vi "SetAttributeViBoolean_SS-DMod_ListSeq_RF.vi"(7 "AttributeValue (Off)":bool, 8 "error in (no error)":errorcluster {"code" format="%.0x"}, 9 "AttributeID":u32(ring)=1150917 items=["SS_DIGITALMODULATION_ARB_ENABLED"=1150917, "SS_DIGITALMODULATION_ARB_EXTERNAL_TRIGGER_DELAY_ENABLED"=1150886, "SS_DIGITALMODULATION_ARB_IQADJUSTMENT_ENABLED"=1150918, "SS_DIGITALMODULATION_ARB_SEQUENCE_SYNC_ENABLED"=1150907, "SS_LISTSEQUENCER_ENABLED"=1150903, "SS_RFGENERATOR_MODULATION_AM_ENABLED"=1150927, "SS_RFGENERATOR_MODULATION_ENABLED"=1150940, "SS_RFGENERATOR_MODULATION_FM_ENABLED"=1150930, "SS_RFGENERATOR_MODULATION_PM_ENABLED"=1150932, "SS_RFGENERATOR_OUTPUT_ENABLED"=1150942, "SS_RFGENERATOR_REFERENCE_FREQUENCY_ENABLED"=1150913, "SS_RFGENERATOR_REFERENCE_POWER_ENABLED"=1150915], 10 "RepCapIdentifier":string, 11 "instrument handle":refnum<k15>) -> (0 "error out":errorcluster {"code" format="%.0x"}, 3 "instrument handle out":refnum<k15>)   [LabVIEW 2009, in "Keysight XSAn.lvlib"]
doc: "Sets a Boolean attribute from the instrument driver.\nThe following Attributes are supported:\n\nSS_DIGITALMODULATION_ARB_ENABLED\nSS_DIGITALMODULATION_ARB_EXTERNAL_TRIGGER_DELAY_ENABLED\nSS_DIGITALMODULATION_ARB_IQADJUSTMENT_ENABLED\nSS_DIGITALMODULATION_ARB_SEQUENCE_SYNC_ENABLED\nSS_LISTSEQUENCER_ENABLED\nSS_RFGENERATOR_MODULATION_AM_ENABLED\nSS_RFGENERATOR_MODULATION_ENABLED\nSS_RFGENERATOR_MODULATION_FM_ENABLED\nSS_RFGENERATOR_MODULATION_PM_ENABLED\nSS_RFGENERATOR_OUTPUT_ENABLED\nSS_RFGENERATOR_REFERENCE_FREQUENCY_ENABLED\nSS_RFGENERATOR_REFERENCE_POWER_ENABLED"
uses:
  <instrlib>/Keysight XSAn/Keysight XSAn.lvlib
  AgXSAn.dll
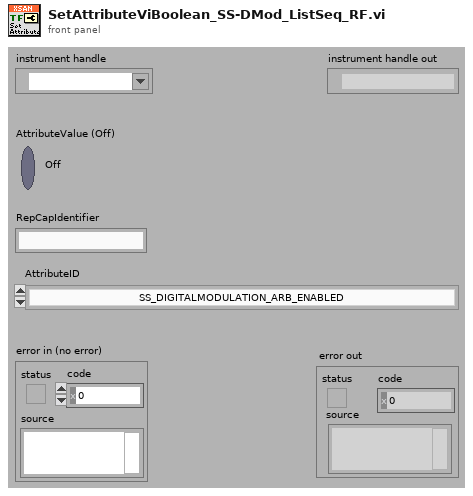
[diagram p1: front panel]
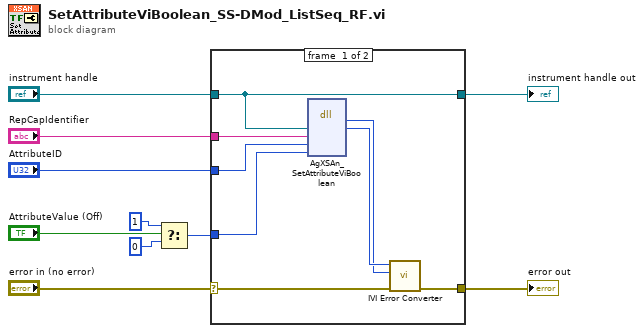
[diagram p0: block diagram]
diagram:
  n1 = Select(t=u16 1, s="AttributeValue (Off)", f=u16 0) -> (s? t:f=w3:u16)
  n2 = case shown="No Error" "error in (no error)" {
    selector: "error in (no error)" -> [w16 w20]
    tunnel: [w15 w20] -> w10
    tunnel: "instrument handle" -> [w11 w19]
    tunnel: "RepCapIdentifier" -> [w14 _]
    tunnel: "AttributeID" -> [w13 _]
    tunnel: w3 -> [w12 _]
    tunnel: [w11 w19] -> w2
    frame #0 {
      n3 = dll-call lib="AgXSAn**.dll" fn="AgXSAn_SetAttributeViBoolean"("Vi"=w11, "RepCapIdentifier"=w14, "AttributeID"=w13, "AttributeValue"=w12) -> ("return type"=w17:i32, "Vi"=w18:u32)  [unwired: 6 in, 2 out]
      n4 = call <instrlib>:"IVI Error Converter.vi"("error in (no error)"=w16, "IVI error code (0)"=w17, "instrument handle"=w18) -> ("error out"=w15:errorcluster)  [unwired: 7 in, 1 out]
    }
    frame #1 {
    }
  }
  "error out" <- w10
  "instrument handle out" <- w2
